vi "输入数据解析.vi"(0 "单个参数补充":dbl, 1 "从板号":dbl=1.0, 2 "主板二维码":string="BNET01", 3 "从板二维码":string="BNET01", 5 "主板引用":refnum<vi>, 7 "从板引用":refnum<vi>, 9 "主板选项":string="三级故障阀值", 11 "枚举":enum16{"主板", "从板"}(ring), 12 "快换":bool caption="快换写入") -> (4 "输出数组":dbl[][](array[numeric]), 6 "数组长度":dbl[](array[numeric]), 8 "循环次数":i32, 10 "命令":u32, 14 "名称":string[](array[string]), 15 "命令序号":u32[](array[numeric]))   [LabVIEW 2013] (continued)
                  disable-tunnel: [w6621 w6626] -> w6616
                  disable-tunnel: w6615 -> [w6620 _]
                  frame Disabled {
                    n2572 = Unbundle By Name(w6620) -> ("整组电压不均衡"=w6619:dbl)
                    n2573 = call "输入分辨率计算-EV05.vi"("1字节?"=FALSE, "数值"=w6619, "偏移量"=0.0, "分辨率"=0.001) -> ("低字节"=w6621:dbl, "高字节1"=w6623:dbl)  [unwired: 1 in, 5 out]
                  }
                  frame Enabled {
                    w6626 = 255 ("高字节1")
                  }
                }
                n2574 = Build Array(w6618, w6616) -> (w6617:i32[])
              }
              frame 7 {
                # "单体电压过高"
                n2575 = disable-structure shown="启用" {
                  disable-tunnel: [w6635 w6638] -> w6630
                  disable-tunnel: [w6633 w6638] -> w6628
                  disable-tunnel: w6627 -> [w6632 _]
                  frame Disabled {
                    n2576 = Unbundle By Name(w6632) -> ("单体电压过高"=w6631:dbl)
                    n2577 = call "输入分辨率计算-EV05.vi"("1字节?"=FALSE, "数值"=w6631, "偏移量"=0.0, "分辨率"=0.001) -> ("低字节"=w6633:dbl, "高字节1"=w6635:dbl)  [unwired: 1 in, 5 out]
                  }
                  frame Enabled {
                    w6638 = 255 ("高字节1")
                  }
                }
                n2578 = Build Array(w6630, w6628) -> (w6629:i32[])
              }
              frame 8 {
                # "单体电压过低"
                n2579 = disable-structure shown="启用" {
                  disable-tunnel: [w6647 w6650] -> w6642
                  disable-tunnel: [w6645 w6650] -> w6640
                  disable-tunnel: w6639 -> [w6644 _]
                  frame Enabled {
                    n2580 = Unbundle By Name(w6644) -> ("单体电压过低"=w6643:dbl)
                    n2581 = call "输入分辨率计算-EV05.vi"("1字节?"=FALSE, "数值"=w6643, "偏移量"=0.0, "分辨率"=0.001) -> ("低字节"=w6645:dbl, "高字节1"=w6647:dbl)  [unwired: 1 in, 5 out]
                  }
                  frame Disabled {
                    w6650 = 255 ("高字节1")
                  }
                }
                n2582 = Build Array(w6642, w6640) -> (w6641:dbl[])
              }
              frame 9 {
                # "充电电流过高"
                n2583 = disable-structure shown="启用" {
                  disable-tunnel: [w6659 w6662] -> w6654
                  disable-tunnel: [w6657 w6662] -> w6652
                  disable-tunnel: w6651 -> [w6656 _]
                  frame Disabled {
                    n2584 = Unbundle By Name(w6656) -> ("充电电流过高"=w6655:dbl)
                    n2585 = call "输入分辨率计算-EV05.vi"("1字节?"=FALSE, "数值"=w6655, "偏移量"=-3000.0, "分辨率"=0.1) -> ("低字节"=w6657:dbl, "高字节1"=w6659:dbl)  [unwired: 1 in, 5 out]
                  }
                  frame Enabled {
                    w6662 = 255 ("高字节1")
                  }
                }
                n2586 = Build Array(w6654, w6652) -> (w6653:i32[])
              }
              frame 10 {
                # "放电电流过高"
                n2587 = disable-structure shown="启用" {
                  disable-tunnel: [w6671 w6674] -> w6666
                  disable-tunnel: [w6669 w6674] -> w6664
                  disable-tunnel: w6663 -> [w6668 _]
                  frame Disabled {
                    n2588 = Unbundle By Name(w6668) -> ("放电电流过高"=w6667:dbl)
                    n2589 = call "输入分辨率计算-EV05.vi"("1字节?"=FALSE, "数值"=w6667, "偏移量"=-3000.0, "分辨率"=0.1) -> ("低字节"=w6669:dbl, "高字节1"=w6671:dbl)  [unwired: 1 in, 5 out]
                  }
                  frame Enabled {
                    w6674 = 255 ("高字节1")
                  }
                }
                n2590 = Build Array(w6666, w6664) -> (w6665:i32[])
              }
              frame 11 {
                # "单组温度不均衡"
                n2591 = disable-structure shown="启用" {
                  disable-tunnel: [w6681 255 ("高字节1")] -> w6677
                  disable-tunnel: w6675 -> [w6679 _]
                  frame Disabled {
                    n2592 = Unbundle By Name(w6679) -> ("单组温度不均衡"=w6678:dbl)
                    n2593 = call "输入分辨率计算-EV05.vi"("1字节?"=TRUE, "数值"=w6678, "偏移量"=0.0, "分辨率"=1.0) -> ("高字节1"=w6681:dbl)  [unwired: 1 in, 6 out]
                  }
                  frame Enabled {
                  }
                }
                n2594 = Build Array(w6677) -> (w6676:i32[])
              }
              frame 12 {
                # "SOC过高"
                n2595 = Unbundle By Name(w6689) -> ("SOC过高"=w6688:dbl)
                n2596 = call "输入分辨率计算-EV05.vi"("1字节?"=FALSE, "数值"=w6688, "偏移量"=0.0, "分辨率"=0.1) -> ("低字节"=w6690:dbl, "高字节1"=w6691:dbl)  [unwired: 1 in, 5 out]
                n2597 = call "二进制解析-8.6.vi"("索引"=4, "数值"=w6691) -> ("低位子数组"=w6694:i32[])  [unwired: 3 out]
                n2598 = call "二进制解析-8.6.vi"("索引"=4, "数值"=w6690) -> ("低位子数组"=w6686:i32[], "高位子数组"=w6693:i32[])  [unwired: 2 out]
                n2599 = Insert Into Array(array=w6694, new element=w6693) -> (w6692:i32[])  [unwired: 1 in]
                n2600 = call "数值二进制转十进制-8.6.vi"("子数组"=w6692) -> ("十进制数值"=w6687:i32)  [unwired: 4 out]
                n2601 = disable-structure shown="启用" {
                  disable-tunnel: w6687 -> [w6702 _]
                  disable-tunnel: [w6702 255 ("高字节1")] -> w6685
                  disable-tunnel: [w6701 i32[] [] ("低位子数组 26")] -> _
                  disable-tunnel: w6686 -> [w6701 _]
                  frame Disabled {
                  }
                  frame Enabled {
                  }
                }
                n2602 = Build Array(w6685, w6685) -> (w6698:i32[])
              }
              frame 13 {
                # "SOC过低"
                n2603 = Unbundle By Name(w6710) -> ("SOC过低"=w6709:dbl)
                n2604 = call "输入分辨率计算-EV05.vi"("1字节?"=FALSE, "数值"=w6709, "偏移量"=0.0, "分辨率"=0.1) -> ("低字节"=w6707:dbl, "高字节1"=w6708:dbl)  [unwired: 1 in, 5 out]
                n2605 = call "二进制解析-8.6.vi"("索引"=4, "数值"=w6708) -> ("低位子数组"=w6706:i32[])  [unwired: 3 out]
                n2606 = disable-structure shown="启用" {
                  disable-tunnel: w6707 -> [w6717 _]
                  disable-tunnel: [w6717 255 ("高字节1")] -> w6705
                  disable-tunnel: w6706 -> [w6716 _]
                  frame Disabled {
                    (unwired) i32[] [] ("低位子数组 4")
                  }
                  frame Enabled {
                  }
                }
                n2607 = Build Array(w6705, w6705) -> (w6713:i32[])
              }
              frame 14 {
                # "内阻过大"
                n2608 = disable-structure shown="启用" {
                  disable-tunnel: w6721 -> [w6726 _]
                  disable-tunnel: [w6722 255 ("高字节1")] -> w6719
                  frame Disabled {
                    n2609 = Unbundle By Name(w6726) -> ("内阻过大"=w6725:dbl)
                    n2610 = call "输入分辨率计算-EV05.vi"("1字节?"=TRUE, "数值"=w6725, "分辨率"=0.1) -> ("高字节1"=w6722:dbl)  [unwired: 2 in, 6 out]
                  }
                  frame Enabled {
                  }
                }
                n2611 = Build Array(w6719) -> (w6720:i32[])
              }
              frame 15 {
                # "极柱温度过高"
                n2612 = disable-structure shown="启用" {
                  disable-tunnel: w6730 -> [w6736 _]
                  disable-tunnel: [w6732 255 ("高字节1")] -> w6728
                  frame Disabled {
                    n2613 = Unbundle By Name(w6736) -> ("极柱温度过高"=w6735:dbl)
                    n2614 = call "输入分辨率计算-EV05.vi"("1字节?"=TRUE, "数值"=w6735, "偏移量"=-40.0, "分辨率"=1.0) -> ("高字节1"=w6732:dbl)  [unwired: 1 in, 6 out]
                  }
                  frame Enabled {
                  }
                }
                n2615 = Build Array(w6728) -> (w6729:i32[])
              }
              frame 16 {
                # "SOH过低"
                n2616 = disable-structure shown="启用" {
                  disable-tunnel: [w6753 w6761] -> w6740
                  disable-tunnel: w6739 -> [w6750 _]
                  disable-tunnel: [w6742 w6761] -> w6738
                  frame Disabled {
                    n2617 = Unbundle By Name(w6750) -> ("SOH过低"=w6749:dbl)
                    n2618 = call "输入分辨率计算-EV05.vi"("1字节?"=FALSE, "数值"=w6749, "偏移量"=0.0, "分辨率"=0.1) -> ("低字节"=w6751:dbl, "高字节1"=w6752:dbl)  [unwired: 1 in, 5 out]
                    n2619 = call "二进制解析-8.6.vi"("索引"=4, "数值"=w6752) -> ("低位子数组"=w6755:i32[])  [unwired: 3 out]
                    n2620 = call "二进制解析-8.6.vi"("索引"=4, "数值"=w6751) -> ("低位子数组"=w6744:i32[], "高位子数组"=w6754:i32[])  [unwired: 2 out]
                    n2621 = call "二进制解析-8.6.vi"("索引"=4, "数值"=0) -> ("低位子数组"=w6745:i32[])  [unwired: 3 out]
                    n2622 = Insert Into Array(array=w6755, new element=w6754) -> (w6748:i32[])  [unwired: 1 in]
                    n2623 = Insert Into Array(array=w6744, new element=w6745) -> (w6743:i32[])  [unwired: 1 in]
                    n2624 = call "数值二进制转十进制-8.6.vi"("子数组"=w6748) -> ("十进制数值"=w6753:i32)  [unwired: 4 out]
                    n2625 = call "数值二进制转十进制-8.6.vi"("子数组"=w6743) -> ("十进制数值"=w6742:i32)  [unwired: 4 out]
                  }
                  frame Enabled {
                    w6761 = 255 ("高字节1")
                  }
                }
                n2626 = Build Array(w6740, w6738) -> (w6741:i32[])
              }
            }
            n2627 = Insert Into Array(array=w6547, new element=w6548) -> (w6546:dbl[])  [unwired: 1 in]
          }
          n2628 = Build Array(w6543) -> (w6542:dbl[][])
          n2629 = Build Array("一级故障阀值") -> (w6533:string[])
        }
        frame "单体电压过低(2)" {
          n2630 = Unbundle By Name(w6767) -> ("一级故障 2"=w6768:refnum<vi>)
          n2631 = property class="Clust (严格)"(reference=w6768) -> ("Value"=w6766:T4)  [unwired: 1 in, 2 out]
          n2632 = for {
            N: 17 -> [_]
            tunnel: w6766 -> [w6778]
            shift-right: [w6775] -> w6772
            shift-left: dbl[] [] -> [w6776]
            i -> [w6779]
            n2633 = case shown="13" w6779 {
              tunnel: w6778 -> [w6780 w6791 w6802 w6812 w6822 w6832 w6844 w6856 w6868 w6880 w6892 w6904 w6918 w6939 w6950 w6959 w6968]
              tunnel: [w6781 w6792 w6803 w6813 w6823 w6834 w6846 w6858 w6870 w6882 w6894 w6905 w6927 w6942 w6949 w6958 w6970] -> w6777
              frame 0, Default {
                # "总电压过高"
                n2634 = disable-structure shown="启用" {
                  disable-tunnel: [w6787 w6790] -> w6783
                  disable-tunnel: [w6786 w6790] -> w6782
                  disable-tunnel: w6780 -> [w6785 _]
                  frame Disabled {
                    n2635 = Unbundle By Name(w6785) -> ("总电压过高"=w6784:dbl)
                    n2636 = call "输入分辨率计算-EV05.vi"("1字节?"=FALSE, "数值"=w6784, "分辨率"=0.1) -> ("低字节"=w6787:dbl, "高字节1"=w6786:dbl)  [unwired: 2 in, 5 out]
                  }
                  frame Enabled {
                    w6790 = 255 ("高字节1")
                  }
                }
                n2637 = Build Array(w6782, w6783) -> (w6781:i32[])
              }
              frame 1 {
                # "总电压过低"
                n2638 = disable-structure shown="启用" {
                  disable-tunnel: [w6798 w6801] -> w6794
                  disable-tunnel: [w6797 w6801] -> w6793
                  disable-tunnel: w6791 -> [w6796 _]
                  frame Disabled {
                    n2639 = Unbundle By Name(w6796) -> ("总电压过低"=w6795:dbl)
                    n2640 = call "输入分辨率计算-EV05.vi"("1字节?"=FALSE, "数值"=w6795, "分辨率"=0.1) -> ("低字节"=w6798:dbl, "高字节1"=w6797:dbl)  [unwired: 2 in, 5 out]
                  }
                  frame Enabled {
                    w6801 = 255 ("高字节1")
                  }
                }
                n2641 = Build Array(w6793, w6794) -> (w6792:i32[])
              }
              frame 2 {
                # "温度过高"
                n2642 = disable-structure shown="启用" {
                  disable-tunnel: [w6808 255 ("高字节1")] -> w6804
                  disable-tunnel: w6802 -> [w6806 _]
                  frame Disabled {
                    n2643 = Unbundle By Name(w6806) -> ("温度过高"=w6805:dbl)
                    n2644 = call "输入分辨率计算-EV05.vi"("1字节?"=TRUE, "数值"=w6805, "偏移量"=-40.0, "分辨率"=1.0) -> ("高字节1"=w6808:dbl)  [unwired: 1 in, 6 out]
                  }
                  frame Enabled {
                  }
                }
                n2645 = Build Array(w6804) -> (w6803:i32[])
              }
              frame 3 {
                # "温度过低"
                n2646 = disable-structure shown="启用" {
                  disable-tunnel: [w6818 255 ("高字节1")] -> w6814
                  disable-tunnel: w6812 -> [w6816 _]
                  frame Disabled {
                    n2647 = Unbundle By Name(w6816) -> ("温度过低"=w6815:dbl)
                    n2648 = call "输入分辨率计算-EV05.vi"("1字节?"=TRUE, "数值"=w6815, "偏移量"=-40.0, "分辨率"=1.0) -> ("高字节1"=w6818:dbl)  [unwired: 1 in, 6 out]
                  }
                  frame Enabled {
                  }
                }
                n2649 = Build Array(w6814) -> (w6813:i32[])
              }
              frame 4 {
                # "整组温度不均衡"
                n2650 = disable-structure shown="启用" {
                  disable-tunnel: [w6828 255 ("高字节1")] -> w6824
                  disable-tunnel: w6822 -> [w6826 _]
                  frame Disabled {
                    n2651 = Unbundle By Name(w6826) -> ("整组温度不均衡"=w6825:dbl)
                    n2652 = call "输入分辨率计算-EV05.vi"("1字节?"=TRUE, "数值"=w6825, "偏移量"=0.0, "分辨率"=1.0) -> ("高字节1"=w6828:dbl)  [unwired: 1 in, 6 out]
                  }
                  frame Enabled {
                  }
                }
                n2653 = Build Array(w6824) -> (w6823:i32[])
              }
              frame 5 {
                # "单组电压不均衡"
                n2654 = disable-structure shown="启用" {
                  disable-tunnel: [w6840 w6843] -> w6835
                  disable-tunnel: [w6838 w6843] -> w6833
                  disable-tunnel: w6832 -> [w6837 _]
                  frame Disabled {
                    n2655 = Unbundle By Name(w6837) -> ("单组电压不均衡"=w6836:dbl)
                    n2656 = call "输入分辨率计算-EV05.vi"("1字节?"=FALSE, "数值"=w6836, "偏移量"=0.0, "分辨率"=0.001) -> ("低字节"=w6838:dbl, "高字节1"=w6840:dbl)  [unwired: 1 in, 5 out]
                  }
                  frame Enabled {
                    w6843 = 255 ("高字节1")
                  }
                }
                n2657 = Build Array(w6835, w6833) -> (w6834:i32[])
              }
              frame 6 {
                # "整组电压不均衡"
                n2658 = disable-structure shown="启用" {
                  disable-tunnel: [w6852 w6855] -> w6847
                  disable-tunnel: [w6850 w6855] -> w6845
                  disable-tunnel: w6844 -> [w6849 _]
                  frame Disabled {
                    n2659 = Unbundle By Name(w6849) -> ("整组电压不均衡"=w6848:dbl)
                    n2660 = call "输入分辨率计算-EV05.vi"("1字节?"=FALSE, "数值"=w6848, "偏移量"=0.0, "分辨率"=0.001) -> ("低字节"=w6850:dbl, "高字节1"=w6852:dbl)  [unwired: 1 in, 5 out]
                  }
                  frame Enabled {
                    w6855 = 255 ("高字节1")
                  }
                }
                n2661 = Build Array(w6847, w6845) -> (w6846:i32[])
              }
              frame 7 {
                # "单体电压过高"
                n2662 = disable-structure shown="启用" {
                  disable-tunnel: [w6864 w6867] -> w6859
                  disable-tunnel: [w6862 w6867] -> w6857
                  disable-tunnel: w6856 -> [w6861 _]
                  frame Disabled {
                    n2663 = Unbundle By Name(w6861) -> ("单体电压过高"=w6860:dbl)
                    n2664 = call "输入分辨率计算-EV05.vi"("1字节?"=FALSE, "数值"=w6860, "偏移量"=0.0, "分辨率"=0.001) -> ("低字节"=w6862:dbl, "高字节1"=w6864:dbl)  [unwired: 1 in, 5 out]
                  }
                  frame Enabled {
                    w6867 = 255 ("高字节1")
                  }
                }
                n2665 = Build Array(w6859, w6857) -> (w6858:i32[])
              }
              frame 8 {
                # "单体电压过低"
                n2666 = disable-structure shown="启用" {
                  disable-tunnel: [w6876 w6879] -> w6871
                  disable-tunnel: [w6874 w6879] -> w6869
                  disable-tunnel: w6868 -> [w6873 _]
                  frame Enabled {
                    n2667 = Unbundle By Name(w6873) -> ("单体电压过低"=w6872:dbl)
                    n2668 = call "输入分辨率计算-EV05.vi"("1字节?"=FALSE, "数值"=w6872, "偏移量"=0.0, "分辨率"=0.001) -> ("低字节"=w6874:dbl, "高字节1"=w6876:dbl)  [unwired: 1 in, 5 out]
                  }
                  frame Disabled {
                    w6879 = 255 ("高字节1")
                  }
                }
                n2669 = Build Array(w6871, w6869) -> (w6870:dbl[])
              }
              frame 9 {
                # "充电电流过高"
                n2670 = disable-structure shown="启用" {
                  disable-tunnel: [w6888 w6891] -> w6883
                  disable-tunnel: [w6886 w6891] -> w6881
                  disable-tunnel: w6880 -> [w6885 _]
                  frame Disabled {
                    n2671 = Unbundle By Name(w6885) -> ("充电电流过高"=w6884:dbl)
                    n2672 = call "输入分辨率计算-EV05.vi"("1字节?"=FALSE, "数值"=w6884, "偏移量"=-3000.0, "分辨率"=0.1) -> ("低字节"=w6886:dbl, "高字节1"=w6888:dbl)  [unwired: 1 in, 5 out]
                  }
                  frame Enabled {
                    w6891 = 255 ("高字节1")
                  }
                }
                n2673 = Build Array(w6883, w6881) -> (w6882:i32[])
              }
              frame 10 {
                # "放电电流过高"
                n2674 = disable-structure shown="启用" {
                  disable-tunnel: [w6900 w6903] -> w6895
                  disable-tunnel: [w6898 w6903] -> w6893
                  disable-tunnel: w6892 -> [w6897 _]
                  frame Disabled {
                    n2675 = Unbundle By Name(w6897) -> ("放电电流过高"=w6896:dbl)
                    n2676 = call "输入分辨率计算-EV05.vi"("1字节?"=FALSE, "数值"=w6896, "偏移量"=-3000.0, "分辨率"=0.1) -> ("低字节"=w6898:dbl, "高字节1"=w6900:dbl)  [unwired: 1 in, 5 out]
                  }
                  frame Enabled {
                    w6903 = 255 ("高字节1")
                  }
                }
                n2677 = Build Array(w6895, w6893) -> (w6894:i32[])
              }
              frame 11 {
                # "单组温度不均衡"
                n2678 = disable-structure shown="启用" {
                  disable-tunnel: [w6910 255 ("高字节1")] -> w6906
                  disable-tunnel: w6904 -> [w6908 _]
                  frame Disabled {
                    n2679 = Unbundle By Name(w6908) -> ("单组温度不均衡"=w6907:dbl)
                    n2680 = call "输入分辨率计算-EV05.vi"("1字节?"=TRUE, "数值"=w6907, "偏移量"=0.0, "分辨率"=1.0) -> ("高字节1"=w6910:dbl)  [unwired: 1 in, 6 out]
                  }
                  frame Enabled {
                  }
                }
                n2681 = Build Array(w6906) -> (w6905:i32[])
              }
              frame 12 {
                # "SOC过高"
                n2682 = Unbundle By Name(w6918) -> ("SOC过高"=w6917:dbl)
                n2683 = call "输入分辨率计算-EV05.vi"("1字节?"=FALSE, "数值"=w6917, "偏移量"=0.0, "分辨率"=0.1) -> ("低字节"=w6919:dbl, "高字节1"=w6920:dbl)  [unwired: 1 in, 5 out]
                n2684 = call "二进制解析-8.6.vi"("索引"=4, "数值"=w6920) -> ("低位子数组"=w6923:i32[])  [unwired: 3 out]
                n2685 = call "二进制解析-8.6.vi"("索引"=4, "数值"=w6919) -> ("低位子数组"=w6915:i32[], "高位子数组"=w6922:i32[])  [unwired: 2 out]
                n2686 = Insert Into Array(array=w6923, new element=w6922) -> (w6921:i32[])  [unwired: 1 in]
                n2687 = call "数值二进制转十进制-8.6.vi"("子数组"=w6921) -> ("十进制数值"=w6916:i32)  [unwired: 4 out]
                n2688 = disable-structure shown="启用" {
                  disable-tunnel: w6916 -> [w6931 _]
                  disable-tunnel: [w6931 255 ("高字节1")] -> w6914
                  disable-tunnel: [w6930 i32[] [] ("低位子数组 26")] -> _
                  disable-tunnel: w6915 -> [w6930 _]
                  frame Disabled {
                  }
                  frame Enabled {
                  }
                }
                n2689 = Build Array(w6914, w6914) -> (w6927:i32[])
              }
              frame 13 {
                # "SOC过低"
                n2690 = Unbundle By Name(w6939) -> ("SOC过低"=w6938:dbl)
                n2691 = call "输入分辨率计算-EV05.vi"("1字节?"=FALSE, "数值"=w6938, "偏移量"=0.0, "分辨率"=0.1) -> ("低字节"=w6936:dbl, "高字节1"=w6937:dbl)  [unwired: 1 in, 5 out]
                n2692 = call "二进制解析-8.6.vi"("索引"=4, "数值"=w6937) -> ("低位子数组"=w6935:i32[])  [unwired: 3 out]
                n2693 = disable-structure shown="启用" {
                  disable-tunnel: w6936 -> [w6946 _]
                  disable-tunnel: [w6946 255 ("高字节1")] -> w6934
                  disable-tunnel: w6935 -> [w6945 _]
                  frame Disabled {
                    (unwired) i32[] [] ("低位子数组 4")
                  }
                  frame Enabled {
                  }
                }
                n2694 = Build Array(w6934, w6934) -> (w6942:i32[])
              }
              frame 14 {
                # "内阻过大"
                n2695 = disable-structure shown="启用" {
                  disable-tunnel: w6950 -> [w6955 _]
                  disable-tunnel: [w6951 255 ("高字节1")] -> w6948
                  frame Disabled {
                    n2696 = Unbundle By Name(w6955) -> ("内阻过大"=w6954:dbl)
                    n2697 = call "输入分辨率计算-EV05.vi"("1字节?"=TRUE, "数值"=w6954, "分辨率"=0.1) -> ("高字节1"=w6951:dbl)  [unwired: 2 in, 6 out]
                  }
                  frame Enabled {
                  }
                }
                n2698 = Build Array(w6948) -> (w6949:i32[])
              }
              frame 15 {
                # "极柱温度过高"
                n2699 = disable-structure shown="启用" {
                  disable-tunnel: w6959 -> [w6965 _]
                  disable-tunnel: [w6961 255 ("高字节1")] -> w6957
                  frame Disabled {
                    n2700 = Unbundle By Name(w6965) -> ("极柱温度过高"=w6964:dbl)
                    n2701 = call "输入分辨率计算-EV05.vi"("1字节?"=TRUE, "数值"=w6964, "偏移量"=-40.0, "分辨率"=1.0) -> ("高字节1"=w6961:dbl)  [unwired: 1 in, 6 out]
                  }
                  frame Enabled {
                  }
                }
                n2702 = Build Array(w6957) -> (w6958:i32[])
              }
              frame 16 {
                # "SOH过低"
                n2703 = disable-structure shown="启用" {
                  disable-tunnel: [w6982 w6990] -> w6969
                  disable-tunnel: w6968 -> [w6979 _]
                  disable-tunnel: [w6971 w6990] -> w6967
                  frame Disabled {
                    n2704 = Unbundle By Name(w6979) -> ("SOH过低"=w6978:dbl)
                    n2705 = call "输入分辨率计算-EV05.vi"("1字节?"=FALSE, "数值"=w6978, "偏移量"=0.0, "分辨率"=0.1) -> ("低字节"=w6980:dbl, "高字节1"=w6981:dbl)  [unwired: 1 in, 5 out]
                    n2706 = call "二进制解析-8.6.vi"("索引"=4, "数值"=w6981) -> ("低位子数组"=w6984:i32[])  [unwired: 3 out]
                    n2707 = call "二进制解析-8.6.vi"("索引"=4, "数值"=w6980) -> ("低位子数组"=w6973:i32[], "高位子数组"=w6983:i32[])  [unwired: 2 out]
                    n2708 = call "二进制解析-8.6.vi"("索引"=4, "数值"=0) -> ("低位子数组"=w6974:i32[])  [unwired: 3 out]
                    n2709 = Insert Into Array(array=w6984, new element=w6983) -> (w6977:i32[])  [unwired: 1 in]
                    n2710 = Insert Into Array(array=w6973, new element=w6974) -> (w6972:i32[])  [unwired: 1 in]
                    n2711 = call "数值二进制转十进制-8.6.vi"("子数组"=w6977) -> ("十进制数值"=w6982:i32)  [unwired: 4 out]
                    n2712 = call "数值二进制转十进制-8.6.vi"("子数组"=w6972) -> ("十进制数值"=w6971:i32)  [unwired: 4 out]
                  }
                  frame Enabled {
                    w6990 = 255 ("高字节1")
                  }
                }
                n2713 = Build Array(w6969, w6967) -> (w6970:i32[])
              }
            }
            n2714 = Insert Into Array(array=w6776, new element=w6777) -> (w6775:dbl[])  [unwired: 1 in]
          }
          n2715 = Build Array(w6772) -> (w6771:dbl[][])
          n2716 = Build Array("二级故障阀值") -> (w6762:string[])
        }
        frame "单体电压过低(3)" {
          n2717 = Unbundle By Name(w6996) -> ("一级故障 3"=w6997:refnum<vi>)
          n2718 = property class="Clust (严格)"(reference=w6997) -> ("Value"=w6995:T4)  [unwired: 1 in, 2 out]
          n2719 = for {
            N: 17 -> [_]
            tunnel: w6995 -> [w7007]
            shift-right: [w7004] -> w7001
            shift-left: dbl[] [] -> [w7005]
            i -> [w7008]
            n2720 = case shown="13" w7008 {
              tunnel: w7007 -> [w7009 w7020 w7031 w7041 w7051 w7061 w7073 w7085 w7097 w7109 w7121 w7133 w7147 w7168 w7179 w7188 w7197]
              tunnel: [w7010 w7021 w7032 w7042 w7052 w7063 w7075 w7087 w7099 w7111 w7123 w7134 w7156 w7171 w7178 w7187 w7199] -> w7006
              frame 0, Default {
                # "总电压过高"
                n2721 = disable-structure shown="启用" {
                  disable-tunnel: [w7016 w7019] -> w7012
                  disable-tunnel: [w7015 w7019] -> w7011
                  disable-tunnel: w7009 -> [w7014 _]
                  frame Disabled {
                    n2722 = Unbundle By Name(w7014) -> ("总电压过高"=w7013:dbl)
                    n2723 = call "输入分辨率计算-EV05.vi"("1字节?"=FALSE, "数值"=w7013, "分辨率"=0.1) -> ("低字节"=w7016:dbl, "高字节1"=w7015:dbl)  [unwired: 2 in, 5 out]
                  }
                  frame Enabled {
                    w7019 = 255 ("高字节1")
                  }
                }
                n2724 = Build Array(w7011, w7012) -> (w7010:i32[])
              }
              frame 1 {
                # "总电压过低"
                n2725 = disable-structure shown="启用" {
                  disable-tunnel: [w7027 w7030] -> w7023
                  disable-tunnel: [w7026 w7030] -> w7022
                  disable-tunnel: w7020 -> [w7025 _]
                  frame Disabled {
                    n2726 = Unbundle By Name(w7025) -> ("总电压过低"=w7024:dbl)
                    n2727 = call "输入分辨率计算-EV05.vi"("1字节?"=FALSE, "数值"=w7024, "分辨率"=0.1) -> ("低字节"=w7027:dbl, "高字节1"=w7026:dbl)  [unwired: 2 in, 5 out]
                  }
                  frame Enabled {
                    w7030 = 255 ("高字节1")
                  }
                }
                n2728 = Build Array(w7022, w7023) -> (w7021:i32[])
              }
              frame 2 {
                # "温度过高"
                n2729 = disable-structure shown="启用" {
                  disable-tunnel: [w7037 255 ("高字节1")] -> w7033
                  disable-tunnel: w7031 -> [w7035 _]
                  frame Disabled {
                    n2730 = Unbundle By Name(w7035) -> ("温度过高"=w7034:dbl)
                    n2731 = call "输入分辨率计算-EV05.vi"("1字节?"=TRUE, "数值"=w7034, "偏移量"=-40.0, "分辨率"=1.0) -> ("高字节1"=w7037:dbl)  [unwired: 1 in, 6 out]
                  }
                  frame Enabled {
                  }
                }
                n2732 = Build Array(w7033) -> (w7032:i32[])
              }
              frame 3 {
                # "温度过低"
                n2733 = disable-structure shown="启用" {
                  disable-tunnel: [w7047 255 ("高字节1")] -> w7043
                  disable-tunnel: w7041 -> [w7045 _]
                  frame Disabled {
                    n2734 = Unbundle By Name(w7045) -> ("温度过低"=w7044:dbl)
                    n2735 = call "输入分辨率计算-EV05.vi"("1字节?"=TRUE, "数值"=w7044, "偏移量"=-40.0, "分辨率"=1.0) -> ("高字节1"=w7047:dbl)  [unwired: 1 in, 6 out]
                  }
                  frame Enabled {
                  }
                }
                n2736 = Build Array(w7043) -> (w7042:i32[])
              }
              frame 4 {
                # "整组温度不均衡"
                n2737 = disable-structure shown="启用" {
                  disable-tunnel: [w7057 255 ("高字节1")] -> w7053
                  disable-tunnel: w7051 -> [w7055 _]
                  frame Disabled {
                    n2738 = Unbundle By Name(w7055) -> ("整组温度不均衡"=w7054:dbl)
                    n2739 = call "输入分辨率计算-EV05.vi"("1字节?"=TRUE, "数值"=w7054, "偏移量"=0.0, "分辨率"=1.0) -> ("高字节1"=w7057:dbl)  [unwired: 1 in, 6 out]
                  }
                  frame Enabled {
                  }
                }
                n2740 = Build Array(w7053) -> (w7052:i32[])
              }
              frame 5 {
                # "单组电压不均衡"
                n2741 = disable-structure shown="启用" {
                  disable-tunnel: [w7069 w7072] -> w7064
                  disable-tunnel: [w7067 w7072] -> w7062
                  disable-tunnel: w7061 -> [w7066 _]
                  frame Disabled {
                    n2742 = Unbundle By Name(w7066) -> ("单组电压不均衡"=w7065:dbl)
                    n2743 = call "输入分辨率计算-EV05.vi"("1字节?"=FALSE, "数值"=w7065, "偏移量"=0.0, "分辨率"=0.001) -> ("低字节"=w7067:dbl, "高字节1"=w7069:dbl)  [unwired: 1 in, 5 out]
                  }
                  frame Enabled {
                    w7072 = 255 ("高字节1")
                  }
                }
                n2744 = Build Array(w7064, w7062) -> (w7063:i32[])
              }
              frame 6 {
                # "整组电压不均衡"
                n2745 = disable-structure shown="启用" {
                  disable-tunnel: [w7081 w7084] -> w7076
                  disable-tunnel: [w7079 w7084] -> w7074
                  disable-tunnel: w7073 -> [w7078 _]
                  frame Disabled {
                    n2746 = Unbundle By Name(w7078) -> ("整组电压不均衡"=w7077:dbl)
                    n2747 = call "输入分辨率计算-EV05.vi"("1字节?"=FALSE, "数值"=w7077, "偏移量"=0.0, "分辨率"=0.001) -> ("低字节"=w7079:dbl, "高字节1"=w7081:dbl)  [unwired: 1 in, 5 out]
                  }
                  frame Enabled {
                    w7084 = 255 ("高字节1")
                  }
                }
                n2748 = Build Array(w7076, w7074) -> (w7075:i32[])
              }
              frame 7 {
                # "单体电压过高"
                n2749 = disable-structure shown="启用" {
                  disable-tunnel: [w7093 w7096] -> w7088
                  disable-tunnel: [w7091 w7096] -> w7086
                  disable-tunnel: w7085 -> [w7090 _]
                  frame Disabled {
                    n2750 = Unbundle By Name(w7090) -> ("单体电压过高"=w7089:dbl)
                    n2751 = call "输入分辨率计算-EV05.vi"("1字节?"=FALSE, "数值"=w7089, "偏移量"=0.0, "分辨率"=0.001) -> ("低字节"=w7091:dbl, "高字节1"=w7093:dbl)  [unwired: 1 in, 5 out]
                  }
                  frame Enabled {
                    w7096 = 255 ("高字节1")
                  }
                }
                n2752 = Build Array(w7088, w7086) -> (w7087:i32[])
              }
              frame 8 {
                # "单体电压过低"
                n2753 = disable-structure shown="启用" {
                  disable-tunnel: [w7105 w7108] -> w7100
                  disable-tunnel: [w7103 w7108] -> w7098
                  disable-tunnel: w7097 -> [w7102 _]
                  frame Enabled {
                    n2754 = Unbundle By Name(w7102) -> ("单体电压过低"=w7101:dbl)
                    n2755 = call "输入分辨率计算-EV05.vi"("1字节?"=FALSE, "数值"=w7101, "偏移量"=0.0, "分辨率"=0.001) -> ("低字节"=w7103:dbl, "高字节1"=w7105:dbl)  [unwired: 1 in, 5 out]
                  }
                  frame Disabled {
                    w7108 = 255 ("高字节1")
                  }
                }
                n2756 = Build Array(w7100, w7098) -> (w7099:dbl[])
              }
              frame 9 {
                # "充电电流过高"
                n2757 = disable-structure shown="启用" {
                  disable-tunnel: [w7117 w7120] -> w7112
                  disable-tunnel: [w7115 w7120] -> w7110
                  disable-tunnel: w7109 -> [w7114 _]
                  frame Disabled {
                    n2758 = Unbundle By Name(w7114) -> ("充电电流过高"=w7113:dbl)
                    n2759 = call "输入分辨率计算-EV05.vi"("1字节?"=FALSE, "数值"=w7113, "偏移量"=-3000.0, "分辨率"=0.1) -> ("低字节"=w7115:dbl, "高字节1"=w7117:dbl)  [unwired: 1 in, 5 out]
                  }
                  frame Enabled {
                    w7120 = 255 ("高字节1")
                  }
                }
                n2760 = Build Array(w7112, w7110) -> (w7111:i32[])
              }
              frame 10 {
                # "放电电流过高"
                n2761 = disable-structure shown="启用" {
                  disable-tunnel: [w7129 w7132] -> w7124
                  disable-tunnel: [w7127 w7132] -> w7122
                  disable-tunnel: w7121 -> [w7126 _]
                  frame Disabled {
                    n2762 = Unbundle By Name(w7126) -> ("放电电流过高"=w7125:dbl)
                    n2763 = call "输入分辨率计算-EV05.vi"("1字节?"=FALSE, "数值"=w7125, "偏移量"=-3000.0, "分辨率"=0.1) -> ("低字节"=w7127:dbl, "高字节1"=w7129:dbl)  [unwired: 1 in, 5 out]
                  }
                  frame Enabled {
                    w7132 = 255 ("高字节1")
                  }
                }
                n2764 = Build Array(w7124, w7122) -> (w7123:i32[])
              }
              frame 11 {
                # "单组温度不均衡"
                n2765 = disable-structure shown="启用" {
                  disable-tunnel: [w7139 255 ("高字节1")] -> w7135
                  disable-tunnel: w7133 -> [w7137 _]
                  frame Disabled {
                    n2766 = Unbundle By Name(w7137) -> ("单组温度不均衡"=w7136:dbl)
                    n2767 = call "输入分辨率计算-EV05.vi"("1字节?"=TRUE, "数值"=w7136, "偏移量"=0.0, "分辨率"=1.0) -> ("高字节1"=w7139:dbl)  [unwired: 1 in, 6 out]
                  }
                  frame Enabled {
                  }
                }
                n2768 = Build Array(w7135) -> (w7134:i32[])
              }
              frame 12 {
                # "SOC过高"
                n2769 = Unbundle By Name(w7147) -> ("SOC过高"=w7146:dbl)
                n2770 = call "输入分辨率计算-EV05.vi"("1字节?"=FALSE, "数值"=w7146, "偏移量"=0.0, "分辨率"=0.1) -> ("低字节"=w7148:dbl, "高字节1"=w7149:dbl)  [unwired: 1 in, 5 out]
                n2771 = call "二进制解析-8.6.vi"("索引"=4, "数值"=w7149) -> ("低位子数组"=w7152:i32[])  [unwired: 3 out]
                n2772 = call "二进制解析-8.6.vi"("索引"=4, "数值"=w7148) -> ("低位子数组"=w7144:i32[], "高位子数组"=w7151:i32[])  [unwired: 2 out]
                n2773 = Insert Into Array(array=w7152, new element=w7151) -> (w7150:i32[])  [unwired: 1 in]
                n2774 = call "数值二进制转十进制-8.6.vi"("子数组"=w7150) -> ("十进制数值"=w7145:i32)  [unwired: 4 out]
                n2775 = disable-structure shown="启用" {
                  disable-tunnel: w7145 -> [w7160 _]
                  disable-tunnel: [w7160 255 ("高字节1")] -> w7143
                  disable-tunnel: [w7159 i32[] [] ("低位子数组 26")] -> _
                  disable-tunnel: w7144 -> [w7159 _]
                  frame Disabled {
                  }
                  frame Enabled {
                  }
                }
                n2776 = Build Array(w7143, w7143) -> (w7156:i32[])
              }
              frame 13 {
                # "SOC过低"
                n2777 = Unbundle By Name(w7168) -> ("SOC过低"=w7167:dbl)
                n2778 = call "输入分辨率计算-EV05.vi"("1字节?"=FALSE, "数值"=w7167, "偏移量"=0.0, "分辨率"=0.1) -> ("低字节"=w7165:dbl, "高字节1"=w7166:dbl)  [unwired: 1 in, 5 out]
                n2779 = call "二进制解析-8.6.vi"("索引"=4, "数值"=w7166) -> ("低位子数组"=w7164:i32[])  [unwired: 3 out]
                n2780 = disable-structure shown="启用" {
                  disable-tunnel: w7165 -> [w7175 _]
                  disable-tunnel: [w7175 255 ("高字节1")] -> w7163
                  disable-tunnel: w7164 -> [w7174 _]
                  frame Disabled {
                    (unwired) i32[] [] ("低位子数组 4")
                  }
                  frame Enabled {
                  }
                }
                n2781 = Build Array(w7163, w7163) -> (w7171:i32[])
              }
              frame 14 {
                # "内阻过大"
                n2782 = disable-structure shown="启用" {
                  disable-tunnel: w7179 -> [w7184 _]
                  disable-tunnel: [w7180 255 ("高字节1")] -> w7177
                  frame Disabled {
                    n2783 = Unbundle By Name(w7184) -> ("内阻过大"=w7183:dbl)
                    n2784 = call "输入分辨率计算-EV05.vi"("1字节?"=TRUE, "数值"=w7183, "分辨率"=0.1) -> ("高字节1"=w7180:dbl)  [unwired: 2 in, 6 out]
                  }
                  frame Enabled {
                  }
                }
                n2785 = Build Array(w7177) -> (w7178:i32[])
              }
              frame 15 {
                # "极柱温度过高"
                n2786 = disable-structure shown="启用" {
                  disable-tunnel: w7188 -> [w7194 _]
                  disable-tunnel: [w7190 255 ("高字节1")] -> w7186
                  frame Disabled {
                    n2787 = Unbundle By Name(w7194) -> ("极柱温度过高"=w7193:dbl)
                    n2788 = call "输入分辨率计算-EV05.vi"("1字节?"=TRUE, "数值"=w7193, "偏移量"=-40.0, "分辨率"=1.0) -> ("高字节1"=w7190:dbl)  [unwired: 1 in, 6 out]
                  }
                  frame Enabled {
                  }
                }
                n2789 = Build Array(w7186) -> (w7187:i32[])
              }
              frame 16 {
                # "SOH过低"
                n2790 = disable-structure shown="启用" {
                  disable-tunnel: [w7211 w7219] -> w7198
                  disable-tunnel: w7197 -> [w7208 _]
                  disable-tunnel: [w7200 w7219] -> w7196
                  frame Disabled {
                    n2791 = Unbundle By Name(w7208) -> ("SOH过低"=w7207:dbl)
                    n2792 = call "输入分辨率计算-EV05.vi"("1字节?"=FALSE, "数值"=w7207, "偏移量"=0.0, "分辨率"=0.1) -> ("低字节"=w7209:dbl, "高字节1"=w7210:dbl)  [unwired: 1 in, 5 out]
                    n2793 = call "二进制解析-8.6.vi"("索引"=4, "数值"=w7210) -> ("低位子数组"=w7213:i32[])  [unwired: 3 out]
                    n2794 = call "二进制解析-8.6.vi"("索引"=4, "数值"=w7209) -> ("低位子数组"=w7202:i32[], "高位子数组"=w7212:i32[])  [unwired: 2 out]
                    n2795 = call "二进制解析-8.6.vi"("索引"=4, "数值"=0) -> ("低位子数组"=w7203:i32[])  [unwired: 3 out]
                    n2796 = Insert Into Array(array=w7213, new element=w7212) -> (w7206:i32[])  [unwired: 1 in]
                    n2797 = Insert Into Array(array=w7202, new element=w7203) -> (w7201:i32[])  [unwired: 1 in]
                    n2798 = call "数值二进制转十进制-8.6.vi"("子数组"=w7206) -> ("十进制数值"=w7211:i32)  [unwired: 4 out]
                    n2799 = call "数值二进制转十进制-8.6.vi"("子数组"=w7201) -> ("十进制数值"=w7200:i32)  [unwired: 4 out]
                  }
                  frame Enabled {
                    w7219 = 255 ("高字节1")
                  }
                }
                n2800 = Build Array(w7198, w7196) -> (w7199:i32[])
              }
            }
            n2801 = Insert Into Array(array=w7005, new element=w7006) -> (w7004:dbl[])  [unwired: 1 in]
          }
          n2802 = Build Array(w7001) -> (w7000:dbl[][])
          n2803 = Build Array("三级故障阀值") -> (w6991:string[])
        }
        frame "充电电流过高" {
          n2804 = Unbundle By Name(w7225) -> ("一级故障"=w7226:refnum<vi>)
          n2805 = property class="Clust (严格)"(reference=w7226) -> ("Value"=w7224:T4)  [unwired: 1 in, 2 out]
          n2806 = for {
            N: 17 -> [_]
            tunnel: w7224 -> [w7236]
            shift-right: [w7233] -> w7230
            shift-left: dbl[] [] -> [w7234]
            i -> [w7237]
            n2807 = case shown="13" w7237 {
              tunnel: w7236 -> [w7238 w7249 w7260 w7270 w7280 w7290 w7302 w7314 w7326 w7338 w7350 w7362 w7376 w7397 w7409 w7418 w7427]
              tunnel: [w7239 w7250 w7261 w7271 w7281 w7292 w7304 w7316 w7328 w7340 w7352 w7363 w7385 w7400 w7408 w7417 w7429] -> w7235
              frame 0, Default {
                # "总电压过高"
                n2808 = disable-structure shown="启用" {
                  disable-tunnel: [w7245 w7248] -> w7241
                  disable-tunnel: [w7244 w7248] -> w7240
                  disable-tunnel: w7238 -> [w7243 _]
                  frame Disabled {
                    n2809 = Unbundle By Name(w7243) -> ("总电压过高"=w7242:dbl)
                    n2810 = call "输入分辨率计算-EV05.vi"("1字节?"=FALSE, "数值"=w7242, "分辨率"=0.1) -> ("低字节"=w7245:dbl, "高字节1"=w7244:dbl)  [unwired: 2 in, 5 out]
                  }
                  frame Enabled {
                    w7248 = 255 ("高字节1")
                  }
                }
                n2811 = Build Array(w7240, w7241) -> (w7239:i32[])
              }
              frame 1 {
                # "总电压过低"
                n2812 = disable-structure shown="启用" {
                  disable-tunnel: [w7256 w7259] -> w7252
                  disable-tunnel: [w7255 w7259] -> w7251
                  disable-tunnel: w7249 -> [w7254 _]
                  frame Disabled {
                    n2813 = Unbundle By Name(w7254) -> ("总电压过低"=w7253:dbl)
                    n2814 = call "输入分辨率计算-EV05.vi"("1字节?"=FALSE, "数值"=w7253, "分辨率"=0.1) -> ("低字节"=w7256:dbl, "高字节1"=w7255:dbl)  [unwired: 2 in, 5 out]
                  }
                  frame Enabled {
                    w7259 = 255 ("高字节1")
                  }
                }
                n2815 = Build Array(w7251, w7252) -> (w7250:i32[])
              }
              frame 2 {
                # "温度过高"
                n2816 = disable-structure shown="启用" {
                  disable-tunnel: [w7266 255 ("高字节1")] -> w7262
                  disable-tunnel: w7260 -> [w7264 _]
                  frame Disabled {
                    n2817 = Unbundle By Name(w7264) -> ("温度过高"=w7263:dbl)
                    n2818 = call "输入分辨率计算-EV05.vi"("1字节?"=TRUE, "数值"=w7263, "偏移量"=-40.0, "分辨率"=1.0) -> ("高字节1"=w7266:dbl)  [unwired: 1 in, 6 out]
                  }
                  frame Enabled {
                  }
                }
                n2819 = Build Array(w7262) -> (w7261:i32[])
              }
              frame 3 {
                # "温度过低"
                n2820 = disable-structure shown="启用" {
                  disable-tunnel: [w7276 255 ("高字节1")] -> w7272
                  disable-tunnel: w7270 -> [w7274 _]
                  frame Disabled {
                    n2821 = Unbundle By Name(w7274) -> ("温度过低"=w7273:dbl)
                    n2822 = call "输入分辨率计算-EV05.vi"("1字节?"=TRUE, "数值"=w7273, "偏移量"=-40.0, "分辨率"=1.0) -> ("高字节1"=w7276:dbl)  [unwired: 1 in, 6 out]
                  }
                  frame Enabled {
                  }
                }
                n2823 = Build Array(w7272) -> (w7271:i32[])
              }
              frame 4 {
                # "整组温度不均衡"
                n2824 = disable-structure shown="启用" {
                  disable-tunnel: [w7286 255 ("高字节1")] -> w7282
                  disable-tunnel: w7280 -> [w7284 _]
                  frame Disabled {
                    n2825 = Unbundle By Name(w7284) -> ("整组温度不均衡"=w7283:dbl)
                    n2826 = call "输入分辨率计算-EV05.vi"("1字节?"=TRUE, "数值"=w7283, "偏移量"=0.0, "分辨率"=1.0) -> ("高字节1"=w7286:dbl)  [unwired: 1 in, 6 out]
                  }
                  frame Enabled {
                  }
                }
                n2827 = Build Array(w7282) -> (w7281:i32[])
              }
              frame 5 {
                # "单组电压不均衡"
                n2828 = disable-structure shown="启用" {
                  disable-tunnel: [w7298 w7301] -> w7293
                  disable-tunnel: [w7296 w7301] -> w7291
                  disable-tunnel: w7290 -> [w7295 _]
                  frame Disabled {
                    n2829 = Unbundle By Name(w7295) -> ("单组电压不均衡"=w7294:dbl)
                    n2830 = call "输入分辨率计算-EV05.vi"("1字节?"=FALSE, "数值"=w7294, "偏移量"=0.0, "分辨率"=0.001) -> ("低字节"=w7296:dbl, "高字节1"=w7298:dbl)  [unwired: 1 in, 5 out]
                  }
                  frame Enabled {
                    w7301 = 255 ("高字节1")
                  }
                }
                n2831 = Build Array(w7293, w7291) -> (w7292:i32[])
              }
              frame 6 {
                # "整组电压不均衡"
                n2832 = disable-structure shown="启用" {
                  disable-tunnel: [w7310 w7313] -> w7305
                  disable-tunnel: [w7308 w7313] -> w7303
                  disable-tunnel: w7302 -> [w7307 _]
                  frame Disabled {
                    n2833 = Unbundle By Name(w7307) -> ("整组电压不均衡"=w7306:dbl)
                    n2834 = call "输入分辨率计算-EV05.vi"("1字节?"=FALSE, "数值"=w7306, "偏移量"=0.0, "分辨率"=0.001) -> ("低字节"=w7308:dbl, "高字节1"=w7310:dbl)  [unwired: 1 in, 5 out]
                  }
                  frame Enabled {
                    w7313 = 255 ("高字节1")
                  }
                }
                n2835 = Build Array(w7305, w7303) -> (w7304:i32[])
              }
              frame 7 {
                # "单体电压过高"
                n2836 = disable-structure shown="启用" {
                  disable-tunnel: [w7322 w7325] -> w7317
                  disable-tunnel: [w7320 w7325] -> w7315
                  disable-tunnel: w7314 -> [w7319 _]
                  frame Disabled {
                    n2837 = Unbundle By Name(w7319) -> ("单体电压过高"=w7318:dbl)
                    n2838 = call "输入分辨率计算-EV05.vi"("1字节?"=FALSE, "数值"=w7318, "偏移量"=0.0, "分辨率"=0.001) -> ("低字节"=w7320:dbl, "高字节1"=w7322:dbl)  [unwired: 1 in, 5 out]
                  }
                  frame Enabled {
                    w7325 = 255 ("高字节1")
                  }
                }
                n2839 = Build Array(w7317, w7315) -> (w7316:i32[])
              }
              frame 8 {
                # "单体电压过低"
                n2840 = disable-structure shown="启用" {
                  disable-tunnel: [w7334 w7337] -> w7329
                  disable-tunnel: [w7332 w7337] -> w7327
                  disable-tunnel: w7326 -> [w7331 _]
                  frame Disabled {
                    n2841 = Unbundle By Name(w7331) -> ("单体电压过低"=w7330:dbl)
                    n2842 = call "输入分辨率计算-EV05.vi"("1字节?"=FALSE, "数值"=w7330, "偏移量"=0.0, "分辨率"=0.001) -> ("低字节"=w7332:dbl, "高字节1"=w7334:dbl)  [unwired: 1 in, 5 out]
                  }
                  frame Enabled {
                    w7337 = 255 ("高字节1")
                  }
                }
                n2843 = Build Array(w7329, w7327) -> (w7328:i32[])
              }
              frame 9 {
                # "充电电流过高"
                n2844 = disable-structure shown="启用" {
                  disable-tunnel: [w7346 w7349] -> w7341
                  disable-tunnel: [w7344 w7349] -> w7339
                  disable-tunnel: w7338 -> [w7343 _]
                  frame Enabled {
                    n2845 = Unbundle By Name(w7343) -> ("充电电流过高"=w7342:dbl)
                    n2846 = call "输入分辨率计算-EV05.vi"("1字节?"=FALSE, "数值"=w7342, "偏移量"=0.0, "分辨率"=0.1) -> ("低字节"=w7344:dbl, "高字节1"=w7346:dbl)  [unwired: 1 in, 5 out]
                  }
                  frame Disabled {
                    w7349 = 255 ("高字节1")
                  }
                }
                n2847 = Build Array(w7341, w7339) -> (w7340:dbl[])
              }
              frame 10 {
                # "放电电流过高"
                n2848 = disable-structure shown="启用" {
                  disable-tunnel: [w7358 w7361] -> w7353
                  disable-tunnel: [w7356 w7361] -> w7351
                  disable-tunnel: w7350 -> [w7355 _]
                  frame Disabled {
                    n2849 = Unbundle By Name(w7355) -> ("放电电流过高"=w7354:dbl)
                    n2850 = call "输入分辨率计算-EV05.vi"("1字节?"=FALSE, "数值"=w7354, "偏移量"=-3000.0, "分辨率"=0.1) -> ("低字节"=w7356:dbl, "高字节1"=w7358:dbl)  [unwired: 1 in, 5 out]
                  }
                  frame Enabled {
                    w7361 = 255 ("高字节1")
                  }
                }
                n2851 = Build Array(w7353, w7351) -> (w7352:i32[])
              }
              frame 11 {
                # "单组温度不均衡"
                n2852 = disable-structure shown="启用" {
                  disable-tunnel: [w7368 255 ("高字节1")] -> w7364
                  disable-tunnel: w7362 -> [w7366 _]
                  frame Disabled {
                    n2853 = Unbundle By Name(w7366) -> ("单组温度不均衡"=w7365:dbl)
                    n2854 = call "输入分辨率计算-EV05.vi"("1字节?"=TRUE, "数值"=w7365, "偏移量"=0.0, "分辨率"=1.0) -> ("高字节1"=w7368:dbl)  [unwired: 1 in, 6 out]
                  }
                  frame Enabled {
                  }
                }
                n2855 = Build Array(w7364) -> (w7363:i32[])
              }
              frame 12 {
                # "SOC过高"
                n2856 = Unbundle By Name(w7376) -> ("SOC过高"=w7375:dbl)
                n2857 = call "输入分辨率计算-EV05.vi"("1字节?"=FALSE, "数值"=w7375, "偏移量"=0.0, "分辨率"=0.1) -> ("低字节"=w7377:dbl, "高字节1"=w7378:dbl)  [unwired: 1 in, 5 out]
                n2858 = call "二进制解析-8.6.vi"("索引"=4, "数值"=w7378) -> ("低位子数组"=w7381:i32[])  [unwired: 3 out]
                n2859 = call "二进制解析-8.6.vi"("索引"=4, "数值"=w7377) -> ("低位子数组"=w7373:i32[], "高位子数组"=w7380:i32[])  [unwired: 2 out]
                n2860 = Insert Into Array(array=w7381, new element=w7380) -> (w7379:i32[])  [unwired: 1 in]
                n2861 = call "数值二进制转十进制-8.6.vi"("子数组"=w7379) -> ("十进制数值"=w7374:i32)  [unwired: 4 out]
                n2862 = disable-structure shown="启用" {
                  disable-tunnel: w7374 -> [w7389 _]
                  disable-tunnel: [w7389 255 ("高字节1")] -> w7372
                  disable-tunnel: [w7388 i32[] [] ("低位子数组 27")] -> _
                  disable-tunnel: w7373 -> [w7388 _]
                  frame Disabled {
                  }
                  frame Enabled {
                  }
                }
                n2863 = Build Array(w7372, w7372) -> (w7385:i32[])
              }
              frame 13 {
                # "SOC过低"
                n2864 = Unbundle By Name(w7397) -> ("SOC过低"=w7396:dbl)
                n2865 = call "输入分辨率计算-EV05.vi"("1字节?"=FALSE, "数值"=w7396, "偏移量"=0.0, "分辨率"=0.1) -> ("低字节"=w7394:dbl, "高字节1"=w7395:dbl)  [unwired: 1 in, 5 out]
                n2866 = call "二进制解析-8.6.vi"("索引"=4, "数值"=w7395) -> ("低位子数组"=w7393:i32[])  [unwired: 3 out]
                n2867 = disable-structure shown="启用" {
                  disable-tunnel: w7394 -> [w7404 _]
                  disable-tunnel: [w7404 255 ("高字节1")] -> w7392
                  disable-tunnel: w7393 -> [w7403 _]
                  disable-tunnel: [w7403 i32[] [] ("低位子数组")] -> _
                  frame Disabled {
                    (unwired) i32[] [] ("低位子数组 4")
                  }
                  frame Enabled {
                  }
                }
                n2868 = Build Array(w7392, w7392) -> (w7400:i32[])
              }
              frame 14 {
                # "内阻过大"
                n2869 = disable-structure shown="启用" {
                  disable-tunnel: w7409 -> [w7414 _]
                  disable-tunnel: [w7410 255 ("高字节1")] -> w7407
                  frame Disabled {
                    n2870 = Unbundle By Name(w7414) -> ("内阻过大"=w7413:dbl)
                    n2871 = call "输入分辨率计算-EV05.vi"("1字节?"=TRUE, "数值"=w7413, "分辨率"=0.1) -> ("高字节1"=w7410:dbl)  [unwired: 2 in, 6 out]
                  }
                  frame Enabled {
                  }
                }
                n2872 = Build Array(w7407) -> (w7408:i32[])
              }
              frame 15 {
                # "极柱温度过高"
                n2873 = disable-structure shown="启用" {
                  disable-tunnel: w7418 -> [w7424 _]
                  disable-tunnel: [w7420 255 ("高字节1")] -> w7416
                  frame Disabled {
                    n2874 = Unbundle By Name(w7424) -> ("极柱温度过高"=w7423:dbl)
                    n2875 = call "输入分辨率计算-EV05.vi"("1字节?"=TRUE, "数值"=w7423, "偏移量"=-40.0, "分辨率"=1.0) -> ("高字节1"=w7420:dbl)  [unwired: 1 in, 6 out]
                  }
                  frame Enabled {
                  }
                }
                n2876 = Build Array(w7416) -> (w7417:i32[])
              }
              frame 16 {
                # "SOH过低"
                n2877 = disable-structure shown="启用" {
                  disable-tunnel: [w7441 w7449] -> w7428
                  disable-tunnel: w7427 -> [w7438 _]
                  disable-tunnel: [w7430 w7449] -> w7426
                  frame Disabled {
                    n2878 = Unbundle By Name(w7438) -> ("SOH过低"=w7437:dbl)
                    n2879 = call "输入分辨率计算-EV05.vi"("1字节?"=FALSE, "数值"=w7437, "偏移量"=0.0, "分辨率"=0.1) -> ("低字节"=w7439:dbl, "高字节1"=w7440:dbl)  [unwired: 1 in, 5 out]
                    n2880 = call "二进制解析-8.6.vi"("索引"=4, "数值"=w7440) -> ("低位子数组"=w7443:i32[])  [unwired: 3 out]
                    n2881 = call "二进制解析-8.6.vi"("索引"=4, "数值"=w7439) -> ("低位子数组"=w7432:i32[], "高位子数组"=w7442:i32[])  [unwired: 2 out]
                    n2882 = call "二进制解析-8.6.vi"("索引"=4, "数值"=0) -> ("低位子数组"=w7433:i32[])  [unwired: 3 out]
                    n2883 = Insert Into Array(array=w7443, new element=w7442) -> (w7436:i32[])  [unwired: 1 in]
                    n2884 = Insert Into Array(array=w7432, new element=w7433) -> (w7431:i32[])  [unwired: 1 in]
                    n2885 = call "数值二进制转十进制-8.6.vi"("子数组"=w7436) -> ("十进制数值"=w7441:i32)  [unwired: 4 out]
                    n2886 = call "数值二进制转十进制-8.6.vi"("子数组"=w7431) -> ("十进制数值"=w7430:i32)  [unwired: 4 out]
                  }
                  frame Enabled {
                    w7449 = 255 ("高字节1")
                  }
                }
